vi "Collaps.vi"(0 "reference in":refnum<class "PackageNode.lvclass">, 1 "Collaps":bool, 5 "error in (no error)":errorcluster) -> (14 "reference out":refnum<class "PackageNode.lvclass">, 19 "error out":errorcluster)   [LabVIEW 2014, in "PackageNode.lvclass"]
uses:
  <resource>/Framework/Providers/Open_GDS/UML/PackageNode_class/PackageNode.lvclass
  <resource>/Framework/Providers/Open_GDS/UML/AbstractNode_class/AbstractNode.lvclass
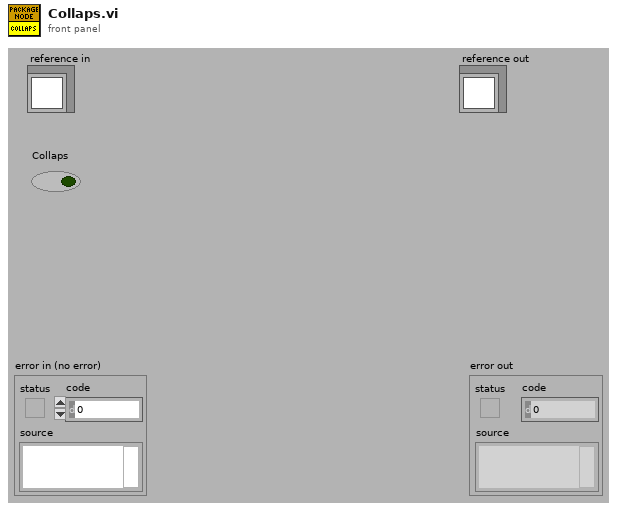
[diagram p1: front panel]
types:
  T1 = typedef "PackageNode.lvclass/ObjectAttributes.ctl" = cluster{"name":string, "contents":refnum<class "MultiLineString.lvclass">, "DEFAULT_TOP_WIDTH":i32, "DEFAULT_TOP_HEIGHT":i32, "DEFAULT_WIDTH":i32, "DEFAULT_HEIGHT":i32, "NAME_GAP":i32, "XGAP":i32, "YGAP":i32, "Collapsed":bool, "Note color":u32, "Justification":u16}
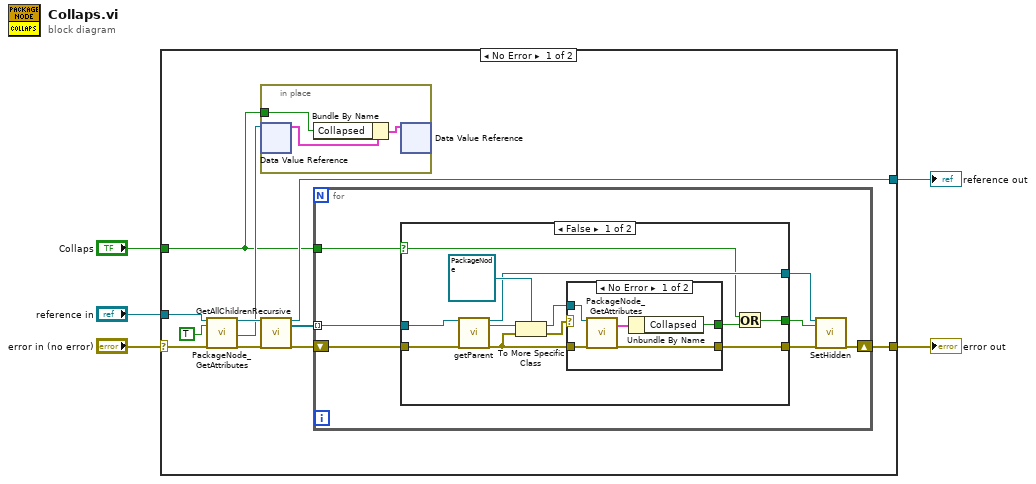
[diagram p0: block diagram]
diagram:
  n1 = case shown="No Error" "error in (no error)" {
    selector: "error in (no error)" -> [w15 w49]
    tunnel: [w14 w49] -> w4
    tunnel: [w13 w48] -> w2
    tunnel: "reference in" -> [w16 w48]
    tunnel: "Collaps" -> [w6 _]
    frame No Error {
      n2 = call <resource>:"PackageNode_GetAttributes.vi"("reference in"=w16, "OnlyGetDvrReference(False)"=TRUE, "error in (no error)"=w15) -> ("reference out"=w12:refnum<class "PackageNode.lvclass">, "DataRef"=w7:refnum<data-value>, "error out"=w9:errorcluster)  [unwired: 13 in, 1 out]
      n3 = in-place {
        in-place-border: w6 -> [w18]
        n4 = in-place-dvr #1(w7) -> (w19:T1)  [unwired: 1 out]
        n5 = Bundle By Name(cluster=w19, "Collapsed"=w18) -> (w17:T1)
        n6 = in-place-dvr #1(w17) -> ()  [unwired: 2 out]
      }
      n7 = call <resource>:"GetAllChildrenRecursive.vi"("reference"=w12, "error in (no error)"=w9) -> ("reference out"=w13:refnum<class "PackageNode.lvclass">, "children"=w11:refnum<class "AbstractNode.lvclass">[], "error out"=w10:errorcluster)  [unwired: 15 in]
      n8 = for {
        tunnel: w11 -> [w24] mode=indexing
        shift-right: [w26] -> w14
        shift-left: w10 -> [w25]
        tunnel: w6 -> [w22]
        n9 = case shown="False" w22 {
          selector: w22 -> [w28 w47]
          tunnel: w25 -> [w38 w46]
          tunnel: w24 -> [w37 w45]
          tunnel: [w33 w46] -> w23
          tunnel: [w32 w45] -> w20
          tunnel: [w27 w47] -> w21
          frame False {
            n10 = call-dynamic "getParent.vi"("reference"=w37, "error in (no error)"=w38) -> ("reference out"=w32:refnum<class "AbstractNode.lvclass">, "parentNode"=w31:refnum<class "AbstractNode.lvclass">, "error out"=w34:errorcluster)  [unwired: 13 in, 2 out]
            n11 = To More Specific Class(target class=refnum<class "PackageNode.lvclass"> refnum ("reference out"), reference=w31, error in=w34) -> (specific class reference=w30:refnum<class "PackageNode.lvclass">, error out=w35:errorcluster)
            n12 = case shown="No Error" w35 {
              tunnel: w34 -> [w43 w44]
              tunnel: [w41 w44] -> w33
              tunnel: w30 -> [w42 _]
              tunnel: [w40 _] -> w29
              frame No Error {
                n13 = call <resource>:"PackageNode_GetAttributes.vi"("reference in"=w42, "error in (no error)"=w43) -> ("Data"=w39:T1, "error out"=w41:errorcluster)  [unwired: 14 in, 2 out]
                n14 = Unbundle By Name(w39) -> ("Collapsed"=w40:bool)
              }
              frame Error {
              }
            }
            n15 = Or(x=w28, y=w29) -> (x .or. y?=w27:bool)
          }
          frame True {
          }
        }
        n16 = call-dynamic "SetHidden.vi"("reference in"=w20, "Hidden"=w21, "error in (no error)"=w23) -> ("error out"=w26:errorcluster)  [unwired: 15 in, 1 out]
      }
    }
    frame Error {
    }
  }
  "error out" <- w4
  "reference out" <- w2
